vi "Agitator Module (Main).vi"(7 "Name of Parent Panel":string="Main.vi", 9 "New Center Coords":T1={"Horizontal"=470, "Vertical"=200}, 10 "Config":variant, 11 "Main UI Message Queue":refnum<queue>) -> ()   [LabVIEW 2018, in "Agitator Module.lvlib"]
doc: "This Continuous Measurement sample project is based on the Queued Message Handler template.\n\nThe Event Handling Loop generates messages based on user interface actions.\n\nThe Message Handling Loop processes messages generated by the Event Handling Loop, or by other messages. There are also Acquisition and Logging message handling loop subVIs, and a chart updating loop."
uses:
  Agitator Module.lvlib
  support/Message Queue/Message Cluster.ctl
  <vilib>/Utility/miscctls.llb/LVPoint32TypeDef.ctl
  controls/UI State.ctl
  Feed Module/Controls/Agitator Module Config Cluster.ctl
  Feed Module/Controls/Agitator Module Settings Cluster.ctl
  IKA EUROSTAR/IKA EUROSTAR Settings.ctl
  Feed Module/Controls/Agitator Module State Cluster.ctl
  Pump Module Folder/Measure Instrument/State Enum.ctl
  Sequencing/Squence Update Cluster.ctl
  Measure Instrument/State Enum.ctl
  Feed Module/Controls/Agitator Module Display.ctl
  support/Message Queue/Enqueue Message (Single).vi
  support/User Event - Stop/User Event - Stop.lvlib
  support/Message Queue/Message Queue.lvlib
  support/Support Library.lvlib
  Measure Instrument/Agitator Module Engine.lvlib
  Agitator Settings Dialog.vi
  support/Command Log VIs/Command Logging.lvlib
  Pump Module Folder/Measure Instrument/Pump Module Engine.lvlib
  Sequencing/Sequencing Library.lvlib
  Measure Instrument/Feed Module Engine.lvlib
  IKA EUROSTAR/IKA EUROSTAR.lvlib
panel:
  in  "Settings Button":bool
  out "H/W":dbl
  out "Original Height":u32
  out "Original Width":u32
  out "RPM":dbl format="%#_5f"
  out "Ring":u16(ring)=2
  out "ScanCode":i16
  out "Log File path":path
  out "Status":string
  in  "Exit":bool
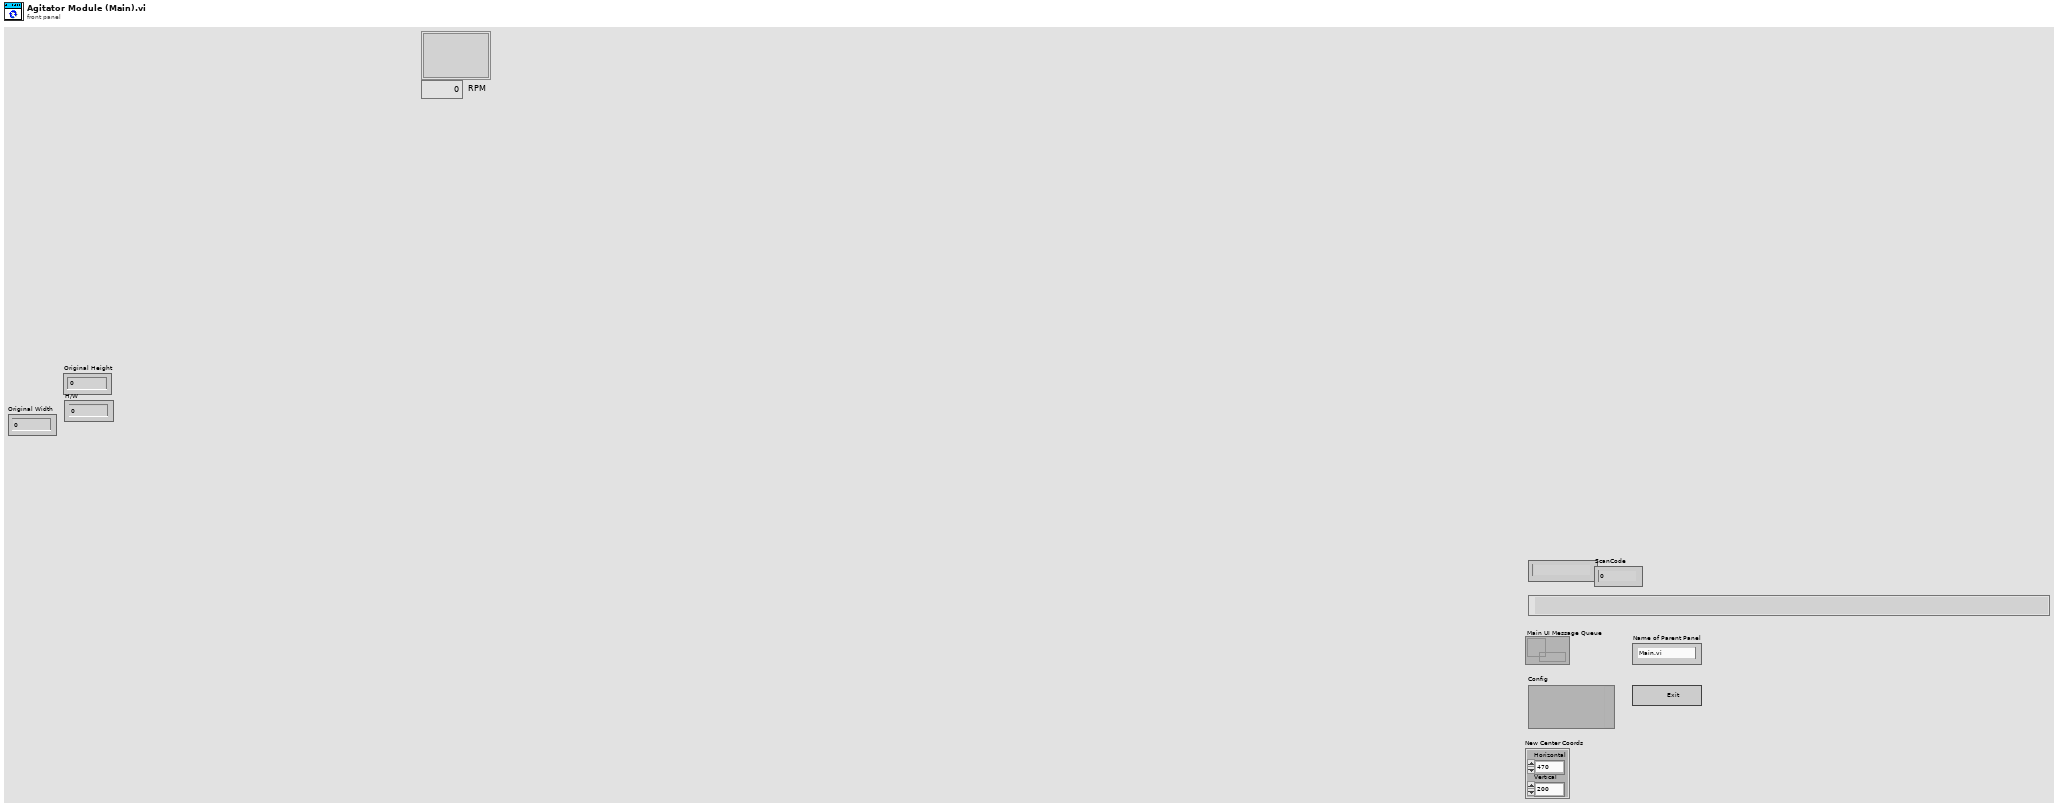
[diagram p1: front panel]
types:
  T1 = typedef "LVPoint32TypeDef.ctl" = cluster{"Horizontal":i32, "Vertical":i32}
  T2 = enum32{"Invalid", "Default", "Floating", "Floating/Auto-Hide", "Modal"}
  T3 = typedef "Agitator Module.lvlib/Agitator Module Config Cluster.ctl" = cluster{"GUID":string, "Drop Coords":T1, "Process Name":string, "User name":string, "Queue Name":string, "Settings":T4, "Load Count":i32}
  T4 = typedef "Agitator Module.lvlib/Agitator Module Settings Cluster.ctl" = cluster{"Cycle Period":dbl, "Agitator Type":string, "Setpoint (µm)":dbl, "IKA EUROSTAR Settings":T5}
  T5 = typedef "IKA EUROSTAR.lvlib/IKA EUROSTAR Settings.ctl" = cluster{"VISA resource name":refnum<visa-resource-name>, "Simulated?":bool}
  T6 = typedef "UI State.ctl" = enum16{"Idle", "Acquiring and Logging", "Waiting for Exit", "Waiting for Exit (Acq Stopped)", "Waiting for Exit (Log Stopped)", "Waiting for Stop", "Waiting for Stop (Acq Stopped)", "Waiting for Stop (Log Stopped)"}
  T7 = typedef "Agitator Module.lvlib/Agitator Module State Cluster.ctl" = cluster{"State":T8, "Start Time":timestamp, "Current Time":timestamp, "Agitator Module Config":T3, "Output Error":bool, "Log Started":bool, "First Iteration":bool, "Data":cluster{"Agitator rpm Value":dbl}, "Agitator On?":enum16{"Off", "On", "Not Initialized", "Over Cutoff"}}
  T8 = typedef "Pump Module.lvlib/Pump Module Engine.lvlib/State Enum.ctl" = enum16{"Measuring", "Idle", "Paused"}
  T9 = typedef "LVPointTypeDef.ctl" = cluster{"Horizontal":i16, "Vertical":i16}
  T10 = typedef "Agitator Module.lvlib/Agitator Message Queues.ctl" = cluster{"Agitator UI":refnum<queue>, "Agitator Engine":refnum<queue>, "Agitator Display":refnum<queue>}
  T11 = typedef "Sequencing Library.lvlib/Squence Update Cluster.ctl" = cluster{"Auto?":bool, "Manual Entry":dbl, "Setpoint":dbl}
  T12 = typedef "Feed Module.lvlib/Feed Module Engine.lvlib/State Enum.ctl" = enum16{"Measuring", "Idle", "Paused"}
  T13 = typedef "Agitator Module.lvlib/Agitator Module Display.ctl" = cluster{"Agitator On?":enum16{"Off", "On", "Not Initialized", "Over Cutoff"}, "Agitator RPM Value":dbl, "Cycle Period":dbl}
  T14 = enum16{"Off", "On", "Not Initialized", "Over Cutoff"}
  T15 = typedef "LVRectTypeDef.ctl" = cluster{"Left":i16, "Top":i16, "Right":i16, "Bottom":i16}
  T16 = cluster{"Shift":bool, "Ctrl":bool, "Alt":bool, "Cmd":bool, "Opt":bool}
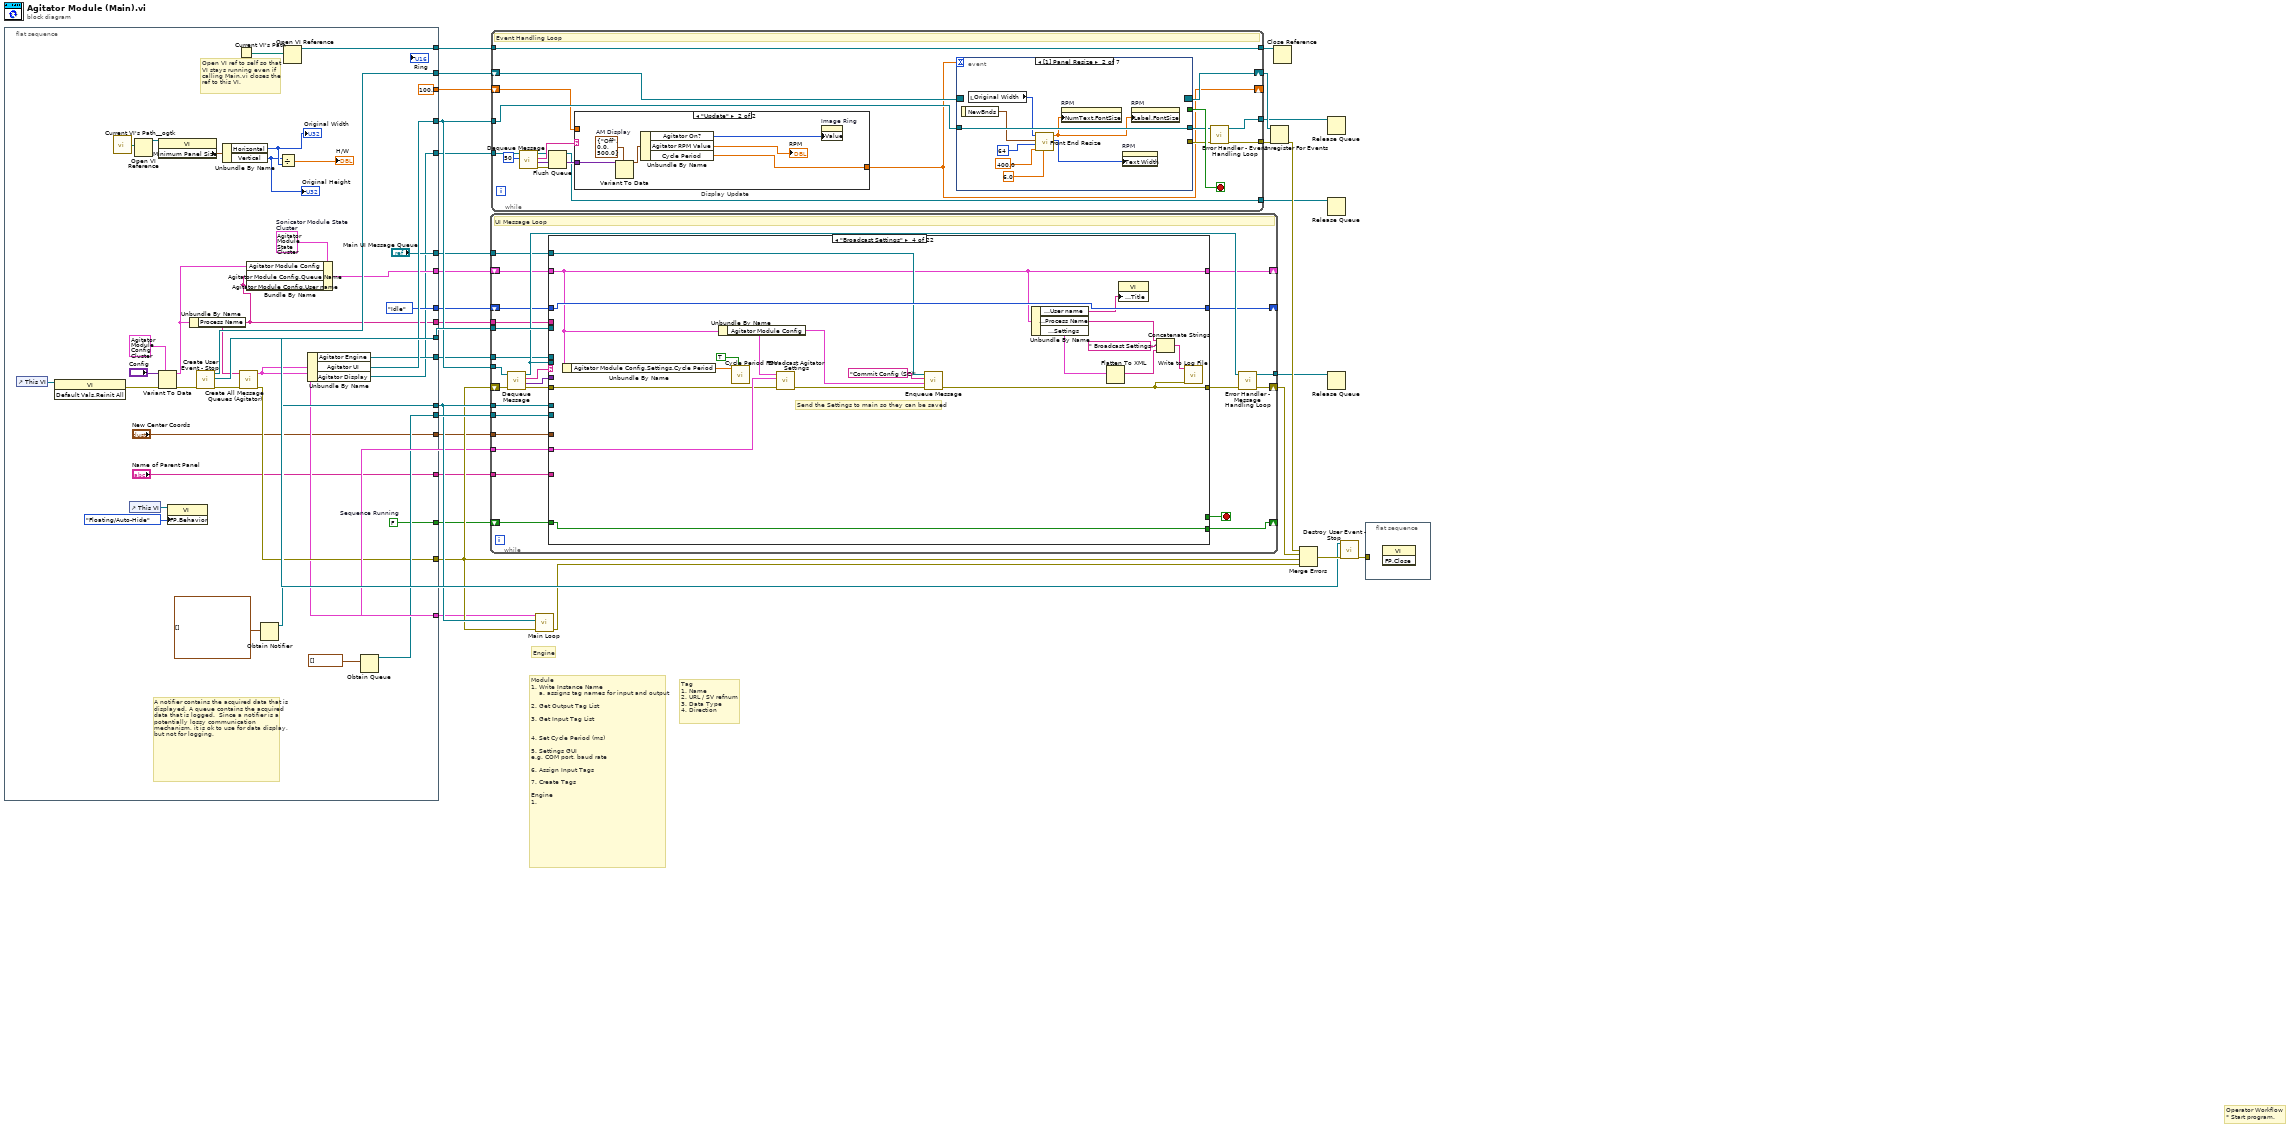
[diagram p0: block diagram]
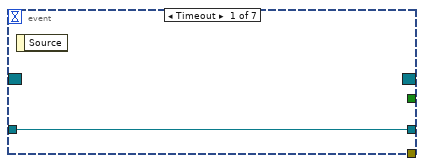
[diagram p3: hidden frame]
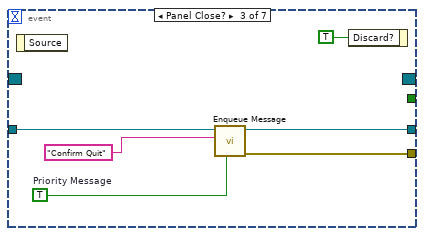
[diagram p4: hidden frame]
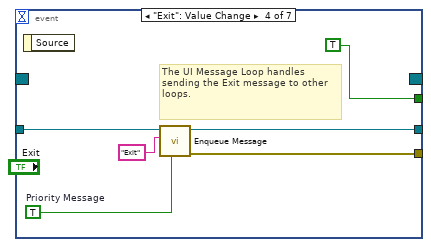
[diagram p5: hidden frame]
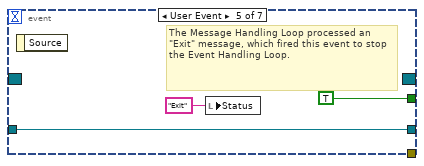
[diagram p6: hidden frame]
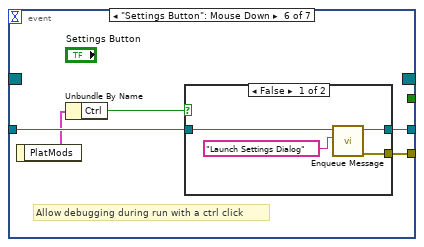
[diagram p7: hidden frame]
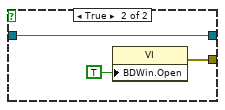
[diagram p8: hidden frame]
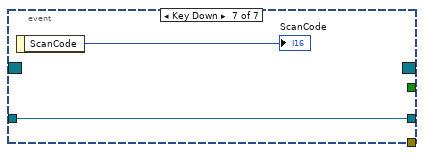
[diagram p9: hidden frame]
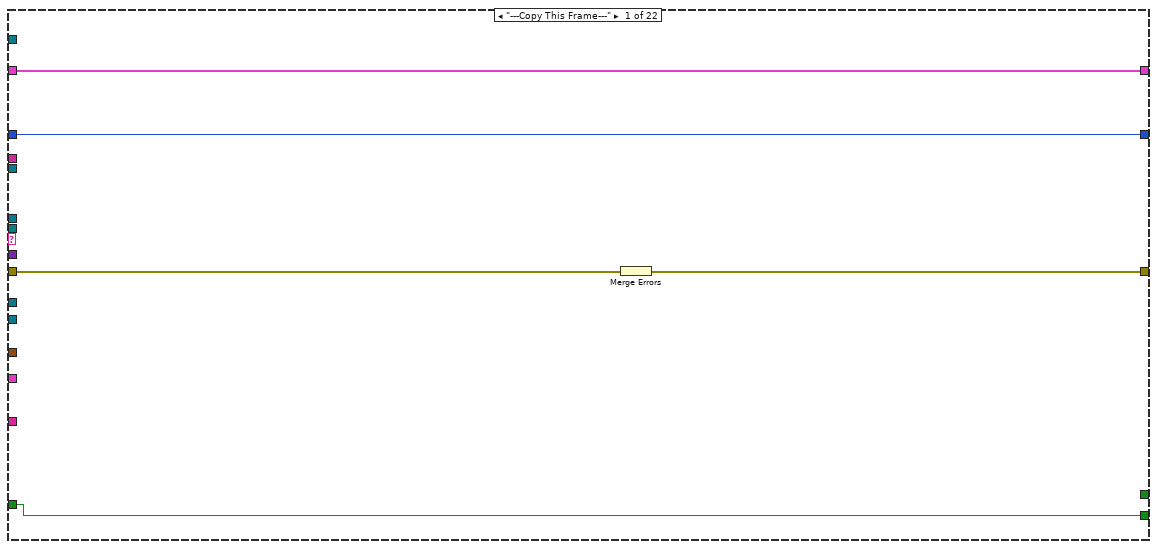
[diagram p10: hidden frame]
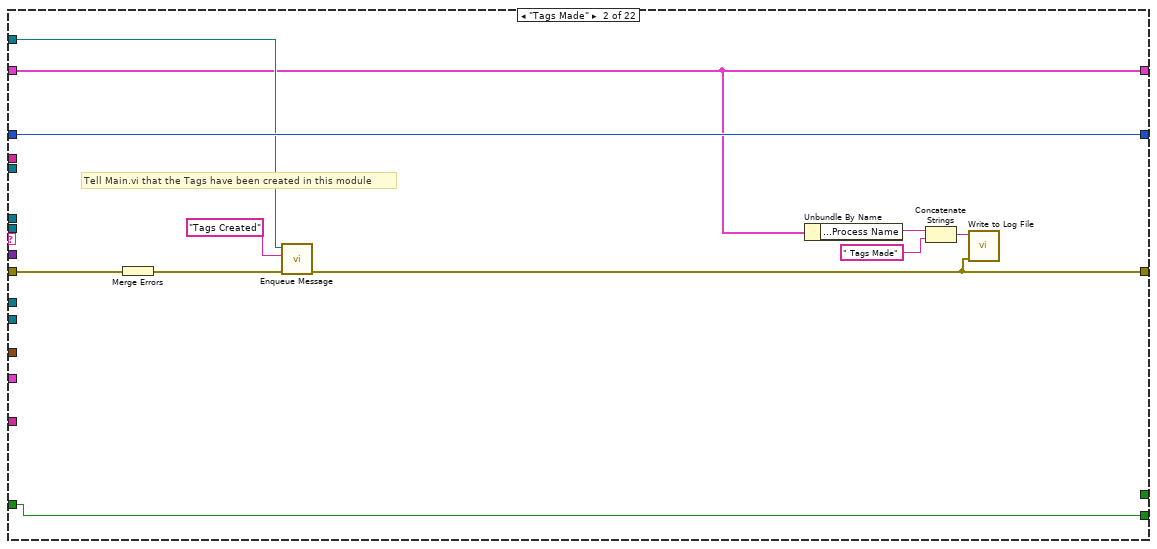
[diagram p11: hidden frame]
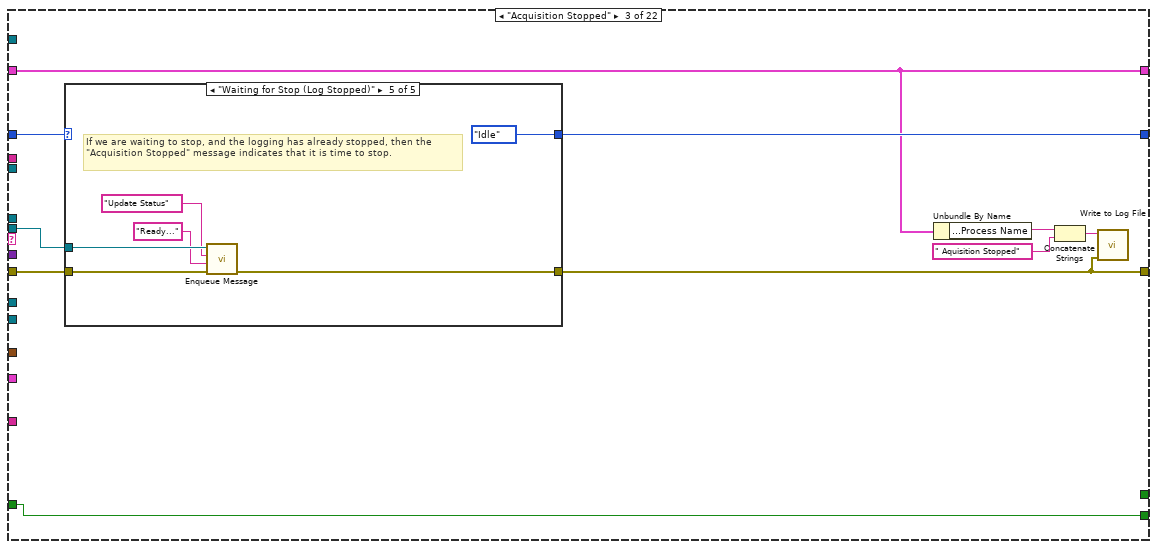
[diagram p12: hidden frame]
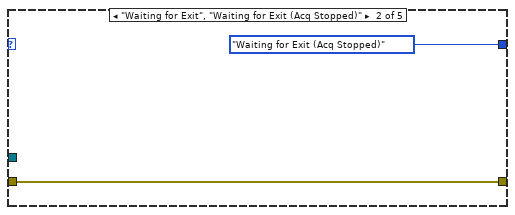
[diagram p14: hidden frame]
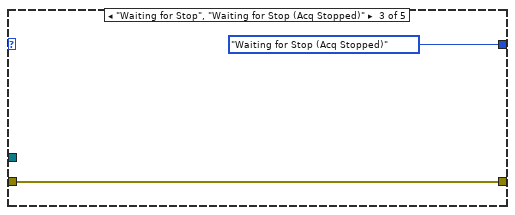
[diagram p15: hidden frame]
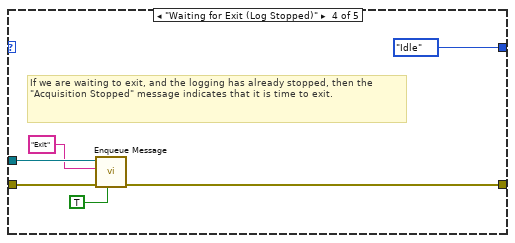
[diagram p16: hidden frame]
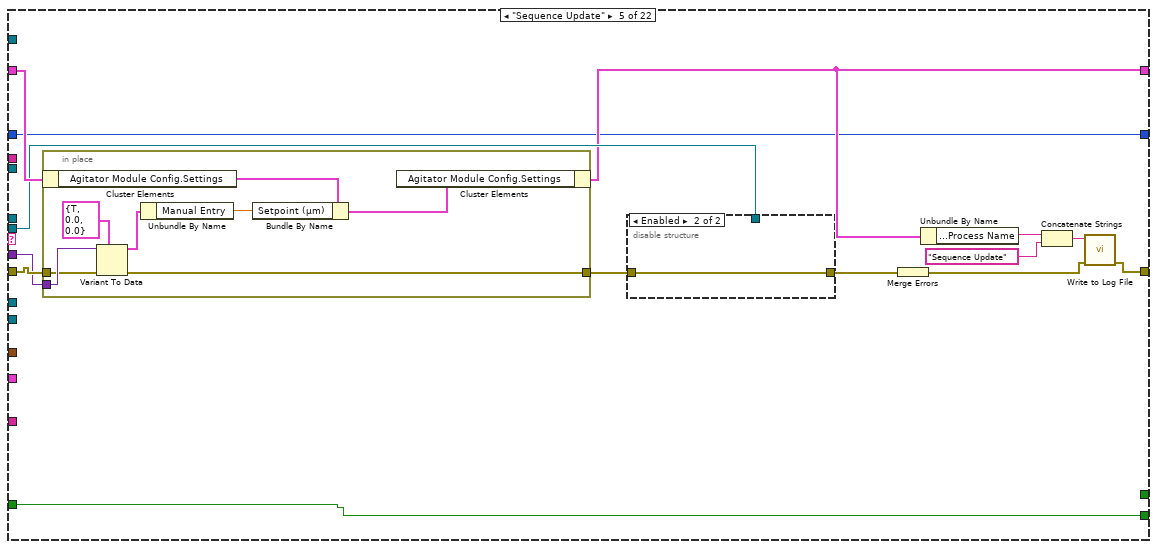
[diagram p17: hidden frame]
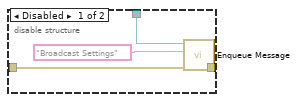
[diagram p18: hidden frame]
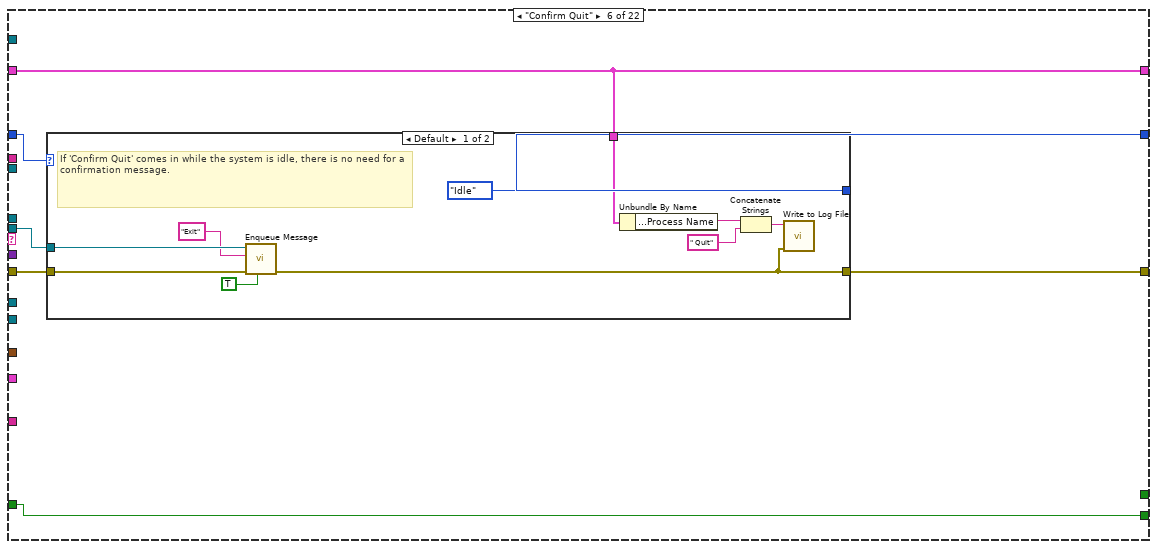
[diagram p19: hidden frame]
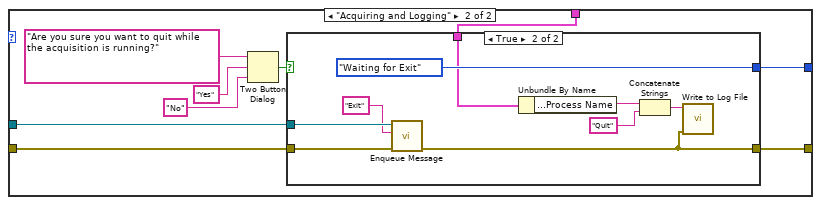
[diagram p20: hidden frame]
diagram:
  # "Engine"
  # "Operator Workflow\n* Start program."
  # "Module \n1. Write Instance Name\n    a. assigns tag names for input and output\n\n2. Get Output Tag List\n\n3. Get Input Tag List\n\n\n4. Set Cycle Period (ms)\n\n5. Settings GUI\ne.g. COM port, baud rate\n\n6. Assign Input Tags\n\n7. Create Tags\n\nEngine\n1."
  # "Tag\n1. Name\n2. URL / SV refnum\n3. Data Type\n4. Direction"
  n1 = flat-sequence {
    tunnel: [w66] -> w26
    tunnel: [w65] -> w25
    tunnel: [w64] -> w22
    tunnel: [UI_State."Idle" ("UI State")] -> w21
    tunnel: [w60] -> w20
    tunnel: [w59] -> w19
    tunnel: [w58] -> w17
    tunnel: [w57] -> w15
    tunnel: [w55] -> w14
    tunnel: ["Main UI Message Queue"] -> w13
    tunnel: [w50] -> w12
    tunnel: [w45] -> w11
    tunnel: [w44] -> w10
    tunnel: ["New Center Coords"] -> w9
    tunnel: ["Name of Parent Panel"] -> w8
    tunnel: [100.0 ("Cycle Period")] -> w6
    tunnel: [w37] -> w2
    tunnel: [w36] -> w1
    frame #0 {
      w37 = FALSE  # Sequence Running
      w51 = T7 {"State"=enum."Idle", "Start Time"=timestamp(0 s since 1904-01-01), "Current Time"=timestamp(0 s since 1904-01-01), "Agitator Module Config"={"GUID"="PID1-Mettler Toledo Scale 1", "Drop Coords"={"Horizontal"=0, "Vertical"=0}, "Process Name"="PID1-Setpoint", "User name"="", "Queue Name"="", "Settings"={"Cycle Period"=500.0, "Agitator Type"="", "Setpoint (µm)"=0.0, "IKA EUROSTAR Settings"={"VISA resource name"="", "Simulated?"=FALSE}}, "Load Count"=0}, "Output Error"=FALSE, "Log Started"=FALSE, "First Iteration"=FALSE, "Data"={"Agitator rpm Value"=0.0}, "Agitator On?"=enum."Off"}  # Sonicator Module State Cluster
      # "Open VI ref to self so that\nVI stays running even if\ncalling Main.vi closes the\nref to this VI."
      # "A notifier contains the acquired data that is displayed. A queue contains the acquired data that is logged.  Since a notifier is a potentially lossy communication mechanism, it is ok to use for data display, but not for logging."
      n2 = control-ref of="This VI"() -> (w48:refnum<vi>)
      n3 = invoke class="VI" method="Default Vals.Reinit All"(reference=w48) -> (error out=w41:errorcluster)  [unwired: 2 in, 2 out]
      n4 = call <userlib>:"Current VI's Path__ogtk.vi"() -> ("Current VI's Path (+ Relative)"=w34:path)  [unwired: 1 in]
      n5 = control-ref of="This VI"() -> (w39:refnum<vi>)
      n6 = Open VI Reference(vi path=w34) -> (vi reference=w33:refnum<vi>)  [unwired: 5 in, 1 out]
      n7 = Variant To Data(error in=w41, type=T3 {"GUID"="", "Drop Coords"={"Horizontal"=0, "Vertical"=0}, "Process Name"="", "User name"="", "Queue Name"="", "Settings"={"Cycle Period"=500.0, "Agitator Type"="", "Setpoint (µm)"=0.0, "IKA EUROSTAR Settings"={"VISA resource name"="", "Simulated?"=FALSE}}, "Load Count"=0} ("Feed Module Config"), Variant="Config") -> (data=w49:T3, error out=w54:errorcluster)
      n8 = property class="VI"(reference=w33) -> ("Minimum Panel Size"=w32:T9)  [unwired: 1 in, 2 out]
      n9 = property class="VI"(reference=w39, "FP.Behavior"=T2."Floating/Auto-Hide" ("Front Panel Window:Behavior")) -> ()  [unwired: 1 in, 2 out]
      n10 = Unbundle By Name(w49) -> ("Process Name"=w36:string)
      n11 = call "Create User Event - Stop.vi"("error in (no error)"=w54) -> ("error out"=w46:errorcluster, "User Event - Stop"=w65:refnum<user-event>, "Stop Event Registration Refnum"=w66:refnum<event-registration>)  [unwired: 8 in]
      n12 = Unbundle By Name(w32) -> ("Horizontal"=w31:i16, "Vertical"=w30:i16)
      "Original Width" <- w31
      "Original Height" <- w30
      n13 = Current VI's Path() -> (path=w56:path)
      n14 = call "Create All Message Queues (Agitator).vi"("error in (no error)"=w46, "Process Name"=w36) -> ("error out"=w45:errorcluster, "Message Queues"=w44:T10)  [unwired: 8 in]
      n15 = Bundle By Name(cluster=w51, "Agitator Module Config"=w49, "Agitator Module Config.Queue Name"=w36, "Agitator Module Config.User name"=w36) -> (w55:T7)
      n16 = Obtain Notifier(notification data type=waveform(dbl)[] []) -> (notifier out=w58:refnum<notifier>)  [unwired: 3 in, 2 out]
      n17 = Divide(x=w30, y=w31) -> (x/y=→"H/W":dbl)
      n18 = Open VI Reference(vi path=w56) -> (vi reference=w57:refnum<vi>)  [unwired: 5 in, 1 out]
      n19 = Unbundle By Name(w44) -> ("Agitator Engine"=w60:refnum<queue>, "Agitator UI"=w64:refnum<queue>, "Agitator Display"=w50:refnum<queue>)
      n20 = Obtain Queue(element data type=waveform(dbl)[] []) -> (queue out=w59:refnum<queue>)  [unwired: 4 in, 2 out]
    }
  }
  n21 = while {
    tunnel: w22 -> [w86]
    tunnel: w25 -> [w90]
    shift-right: [w82] -> w29
    shift-left: w11 -> [w89]
    shift-right: [w73] -> _
    shift-left: w14 -> [w75]
    tunnel: w17 -> [w85]
    tunnel: w19 -> [w84]
    shift-right: [w79] -> _
    shift-left: w21 -> [w80]
    tunnel: w20 -> [w78]
    tunnel: w10 -> [w77]
    tunnel: w13 -> [w74]
    tunnel: w1 -> [w72]
    tunnel: w9 -> [w71]
    tunnel: w8 -> [w70]
    tunnel: [w69] -> w3
    shift-right: [w67] -> _
    shift-left: w2 -> [w68]
    stop <- w91 stop-if-true
    # "UI Message Loop"
    n22 = call "Dequeue Message.vi"("error in (no error)"=w89, "Message Queue"=w86) -> ("error out"=w76:errorcluster, "Message Data"=w87:variant, "Message"=w88:string, "dup Message Queue"=w81:refnum<queue>)  [unwired: 6 in]
    n23 = case "Message Cases" shown="\"Broadcast Settings\"" w88 {
      selector: w88 -> [_ _ _ _ _ _ _ _ _ _ _ _ _ _ _ _ _ _ _ _ _ w470]
      tunnel: w81 -> [_ _ w114 _ w157 w186 _ w238 w253 w276 _ w317 _ w343 _ w383 w387 _ _ w456 _ _]
      tunnel: w76 -> [w96 w107 w115 w149 w161 w185 w221 w233 w257 w275 w302 w313 w333 w344 w368 w382 w388 w411 w425 w451 w466 _]
      tunnel: [w95 w98 w110 w142 w160 w184 w222 w228 w244 w260 w302 w305 w332 w339 w371 w378 w391 w418 w427 w443 w467 w469] -> w83
      tunnel: [_ _ _ _ _ _ _ _ _ TRUE _ _ _ _ _ _ _ _ _ _ _ _] -> w91
      tunnel: w87 -> [_ _ _ _ w158 _ w224 _ w256 w265 _ _ _ _ w369 _ _ _ _ _ w465 _]
      tunnel: w90 -> [_ _ _ _ _ _ _ _ _ w286 _ _ _ _ _ _ _ _ _ _ _ _]
      tunnel: w75 -> [w93 w99 w109 w141 w159 w182 w219 w227 w243 w259 w299 w304 w328 w338 w375 w377 w394 w412 w426 w442 w460 w475]
      tunnel: w85 -> [_ _ _ _ _ _ _ _ _ w284 _ _ _ _ _ _ _ _ _ _ _ _]
      tunnel: w84 -> [_ _ _ _ _ _ _ _ _ w280 _ _ _ _ _ _ _ _ _ _ _ _]
      tunnel: w80 -> [w94 w106 w117 w153 w155 w187 w220 w234 w248 w273 _ _ w334 w346 w374 _ _ _ _ w452 w461 w479]
      tunnel: [w94 w106 w116 w153 w155 w183 w220 w235 w248 w272 UI_State."Idle" ("UI State") UI_State."Idle" ("UI State") w334 w345 w374 UI_State."Acquiring and Logging" ("UI State") UI_State."Acquiring and Logging" ("UI State") UI_State."Acquiring and Logging" ("UI State") UI_State."Acquiring and Logging" ("UI State") w453 w461 w479] -> w79
      tunnel: w78 -> [_ _ _ _ _ _ _ _ _ w279 _ _ _ _ _ _ _ w416 w434 w450 _ _]
      tunnel: w77 -> [_ _ _ w152 _ _ _ _ _ _ _ _ w325 _ _ _ _ _ _ _ _ _]
      tunnel: w74 -> [_ w103 _ w146 _ _ _ _ _ w264 _ _ _ _ _ _ _ _ _ _ _ _]
      tunnel: [w93 w99 w109 w141 w156 w182 w219 w227 w243 w259 w299 w304 w326 w338 w375 w377 w393 w412 w426 w442 w460 w475] -> w73
      tunnel: w72 -> [_ _ _ _ _ _ _ _ _ _ _ w311 _ _ _ _ _ _ _ _ _ _]
      tunnel: w71 -> [_ _ _ _ _ _ _ _ _ _ _ w310 _ _ _ _ _ _ _ _ _ _]
      tunnel: w70 -> [_ _ _ _ _ _ _ _ _ _ _ w309 _ _ _ _ _ _ _ _ _ _]
      tunnel: w68 -> [w92 w97 w108 w137 w154 w181 w218 w226 w241 w258 w298 w303 w327 w337 w365 w376 w389 w410 w424 w441 w459 w468]
      tunnel: [w92 w97 w108 w137 w154 w181 w218 w226 w241 w258 w298 w303 w327 w337 w365 w376 w390 w410 w424 w441 w459 w468] -> w67
      frame "---Copy This Frame---" {
        # "Duplicate this frame when creating new messages.  Change this comment in the duplicated frame to describe this message."
        n24 = Merge Errors(w96) -> (w95:errorcluster)
      }
      frame "Tags Made" {
        # "Tell Main.vi that the Tags have been created in this module"
        # "Duplicate this frame when creating new messages.  Change this comment in the duplicated frame to describe this message."
        n25 = Merge Errors(w107) -> (w104:errorcluster)
        n26 = call-poly "Enqueue Message.vi"("error in (no error)"=w104, "Message"="Tags Created", "Message Queue"=w103) -> ("error out"=w98:errorcluster)  [unwired: 7 in, 1 out]
        n27 = Unbundle By Name(w99) -> ("Agitator Module Config.Process Name"=w102:string)
        n28 = Concatenate Strings(w102, " Tags Made" ("text")) -> (w100:string)
        n29 = call "Write to Log File.vi"("error in"=w98, "text"=w100) -> ()  [unwired: 9 in, 1 out]
      }
      frame "Acquisition Stopped" {
        # "Logic for determining what action to take when the acquisition has stopped."
        n30 = case shown="\"Waiting for Stop (Log Stopped)\"" w117 {
          selector: w117 -> [w119 _ _ _ _]
          tunnel: [w119 UI_State."Waiting for Exit (Acq Stopped)" ("UI State") UI_State."Waiting for Stop (Acq Stopped)" ("UI State") UI_State."Idle" ("UI State") UI_State."Idle" ("UI State")] -> w116
          tunnel: w115 -> [w118 w120 w122 w128 w134]
          tunnel: [w118 w120 w122 w127 w133] -> w110
          tunnel: w114 -> [_ _ _ w126 w132]
          frame Default {
          }
          frame "Waiting for Exit", "Waiting for Exit (Acq Stopped)" {
          }
          frame "Waiting for Stop", "Waiting for Stop (Acq Stopped)" {
          }
          frame "Waiting for Exit (Log Stopped)" {
            # "If we are waiting to exit, and the logging has already stopped, then the \"Acquisition Stopped\" message indicates that it is time to exit."
            n31 = call-poly "Enqueue Message.vi"("Priority Message? (F)"=TRUE, "error in (no error)"=w128, "Message"="Exit", "Message Queue"=w126) -> ("error out"=w127:errorcluster)  [unwired: 6 in, 1 out]
          }
          frame "Waiting for Stop (Log Stopped)" {
            # "If we are waiting to stop, and the logging has already stopped, then the \"Acquisition Stopped\" message indicates that it is time to stop."
            n32 = call-poly "Enqueue Message.vi"("error in (no error)"=w134, "Message Data"="Ready..." ("Message"), "Message"="Update Status", "Message Queue"=w132) -> ("error out"=w133:errorcluster)  [unwired: 6 in, 1 out]
          }
        }
        n33 = Unbundle By Name(w109) -> ("Agitator Module Config.Process Name"=w113:string)
        n34 = Concatenate Strings(w113, " Aquisition Stopped" ("text")) -> (w111:string)
        n35 = call "Write to Log File.vi"("error in"=w110, "text"=w111) -> ()  [unwired: 9 in, 1 out]
      }
      frame "Broadcast Settings" {
        # "Send the Settings to main so they can be saved"
        # "Send the 'Update Settings' message to the Logging and Acquisition message loops."
        n36 = Unbundle By Name(w141) -> ("Agitator Module Config.Settings.Cycle Period"=w150:dbl)
        n37 = Unbundle By Name(w141) -> ("Agitator Module Config"=w145:T3)
        n38 = call "Cycle Period FGV.vi"("Write"=TRUE, "Cycle Period In (ms)"=w150) -> ()  [unwired: 8 in, 2 out]
        n39 = call "Broadcast Agitator Settings.vi"("error in (no error)"=w149, "Message Queues"=w152, "Agitator Module Config"=w145) -> ("error out"=w147:errorcluster)  [unwired: 8 in]
        n40 = call-poly "Enqueue Message.vi"("error in (no error)"=w147, "Message Data"=w145, "Message"="Commit Config (SC)", "Message Queue"=w146) -> ("error out"=w142:errorcluster)  [unwired: 6 in, 1 out]
        n41 = Unbundle By Name(w141) -> ("Agitator Module Config.User name"=w136:string, "Agitator Module Config.Process Name"=w138:string, "Agitator Module Config.Settings"=w140:T4)
        n42 = Flatten To XML(anything=w140) -> (xml string=w139:string)
        n43 = property class="VI"("Front Panel.Title"=w136) -> ()  [unwired: 2 in, 2 out]
        n44 = Concatenate Strings(w138, " Broadcast Settings: " ("text"), w139) -> (w143:string)
        n45 = call "Write to Log File.vi"("error in"=w142, "text"=w143) -> ()  [unwired: 9 in, 1 out]
      }
      frame "Sequence Update" {
        n46 = in-place {
          in-place-border: w158 -> [w177]
          in-place-border: w161 -> [w176]
          in-place-border: [w175] -> w166
          n47 = in-place-cluster #1(w159) -> ("Agitator Module Config.Settings"=w173:T4)
          n48 = Variant To Data(error in=w176, type=T11 {"Auto?"=TRUE, "Manual Entry"=0.0, "Setpoint"=0.0} ("Cluster"), Variant=w177) -> (data=w179:T11, error out=w175:errorcluster)
          n49 = Unbundle By Name(w179) -> ("Manual Entry"=w178:dbl)
          n50 = Bundle By Name(cluster=w173, "Setpoint (µm)"=w178) -> (w174:T4)
          n51 = in-place-cluster #1("Agitator Module Config.Settings"=w174) -> (w156:T7)
        }
        n52 = disable-structure shown="Enabled" {
          disable-tunnel: [w171 w172] -> w167
          disable-tunnel: w157 -> [w169 _]
          disable-tunnel: w166 -> [w168 w172]
          frame Disabled {
            n53 = call-poly "Enqueue Message.vi"("error in (no error)"=w168, "Message"="Broadcast Settings", "Message Queue"=w169) -> ("error out"=w171:errorcluster)  [unwired: 7 in, 1 out]
          }
          frame Enabled {
          }
        }
        n54 = Merge Errors(w167) -> (w163:errorcluster)
        n55 = Unbundle By Name(w156) -> ("Agitator Module Config.Process Name"=w165:string)
        n56 = Concatenate Strings(w165, "Sequence Update" ("text")) -> (w162:string)
        n57 = call "Write to Log File.vi"("error in"=w163, "text"=w162) -> ("error out"=w160:errorcluster)  [unwired: 9 in]
      }
      frame "Confirm Quit" {
        # "Confirm Quit - Message that can confirm whether or not the user wants to exit the application."
        n58 = case shown="Default" w187 {
          tunnel: w186 -> [w196 w203]
          tunnel: w185 -> [w195 w201]
          tunnel: [w189 w200] -> w184
          tunnel: [UI_State."Idle" ("UI State") w199] -> w183
          tunnel: w182 -> [w188 w198]
          frame Default {
            # "If 'Confirm Quit' comes in while the system is idle, there is no need for a confirmation message."
            n59 = call-poly "Enqueue Message.vi"("Priority Message? (F)"=TRUE, "error in (no error)"=w195, "Message"="Exit", "Message Queue"=w196) -> ("error out"=w189:errorcluster)  [unwired: 6 in, 1 out]
            n60 = Unbundle By Name(w188) -> ("Agitator Module Config.Process Name"=w192:string)
            n61 = Concatenate Strings(w192, " Quit" ("text")) -> (w190:string)
            n62 = call "Write to Log File.vi"("error in"=w189, "text"=w190) -> ()  [unwired: 9 in, 1 out]
          }
          frame "Acquiring and Logging" {
            n63 = Two Button Dialog(message="Are you sure you want to quit while the acquisition is running?" ("Confirm Quit Message"), 1:"No" ("No"), 2:"Yes" ("Yes")) -> (T button?=w202:bool)
            n64 = case shown="True" w202 {
              tunnel: w203 -> [_ w217]
              tunnel: w201 -> [w207 w216]
              tunnel: [w207 w210] -> w200
              tunnel: [UI_State."Acquiring and Logging" ("UI State") UI_State."Waiting for Exit" ("UI State")] -> w199
              tunnel: w198 -> [_ w209]
              frame False {
                # "User did not want to quit."
              }
              frame True {
                n65 = call-poly "Enqueue Message.vi"("error in (no error)"=w216, "Message"="Exit", "Message Queue"=w217) -> ("error out"=w210:errorcluster)  [unwired: 7 in, 1 out]
                n66 = Unbundle By Name(w209) -> ("Agitator Module Config.Process Name"=w213:string)
                n67 = Concatenate Strings(w213, "Quit" ("text")) -> (w211:string)
                n68 = call "Write to Log File.vi"("error in"=w210, "text"=w211) -> ()  [unwired: 9 in, 1 out]
              }
            }
          }
        }
      }
      frame "Display Log File Path" {
        n69 = Variant To Data(error in=w221, type=path "", Variant=w224) -> (data=→"Log File path":path, error out=w222:errorcluster)
      }
      frame "E-Stop" {
        # "E-Stop has no effect on the scale"
        # "Message Acquisition and Logging loops to stop"
        # "Stop the pumps."
        n70 = call-poly "Enqueue Message.vi"("error in (no error)"=w233, "Message Data"="Ready..." ("Ready..."), "Message"="Update Status", "Message Queue"=w238) -> ("error out"=w232:errorcluster)  [unwired: 6 in, 1 out]
        n71 = case shown="\"Waiting for Exit\"" w234 {
          selector: w234 -> [_ w240]
          tunnel: [UI_State."Waiting for Stop" ("UI State") w240] -> w235
          frame Default {
          }
          frame "Waiting for Exit" {
          }
        }
        n72 = Merge Errors(w232) -> (w228:errorcluster)
        n73 = Unbundle By Name(w227) -> ("Agitator Module Config.Process Name"=w231:string)
        n74 = Concatenate Strings(w231, " E-STOP" ("text")) -> (w229:string)
        n75 = call "Write to Log File.vi"("error in"=w228, "text"=w229) -> ()  [unwired: 9 in, 1 out]
      }
      frame "Error" {
        # "Error - Check the error message data and respond accordingly. This message is sent by the \"Error Handler\" VIs at the end of each loop in this application."
        n76 = Variant To Data(error in=w257, type=errorcluster {"status"=FALSE, "code"=0, "source"=""} ("error out"), Variant=w256) -> (data=w254:errorcluster, error out=w250:errorcluster)
        n77 = call <vilib>:"General Error Handler.vi"("error in (no error)"=w254) -> ("message"=w242:string)  [unwired: 10 in, 4 out]
        n78 = call-poly "Enqueue Message.vi"("Priority Message? (F)"=TRUE, "Message"="Exit", "Message Queue"=w253) -> ("error out"=w249:errorcluster)  [unwired: 7 in, 1 out]
        n79 = Merge Errors(w249, w250) -> (w244:errorcluster)
        n80 = Unbundle By Name(w243) -> ("Agitator Module Config.Process Name"=w247:string)
        n81 = Concatenate Strings(w247, " Error: " ("text"), w242) -> (w245:string)
        n82 = call "Write to Log File.vi"("error in"=w244, "text"=w245) -> ()  [unwired: 9 in, 1 out]
      }
      frame "Exit" {
        w268 = TRUE  # Delete Module?
        # "Don't check the error outs. The acquisition and logging queues may have already been released."
        # "Close references owned by the Main VI."
        # "Stop the VI"
        # "Exit - Fire the User Event to stop the Event Handling Loop.  Also send Exit messages to the Acquisition and Logging loops."
        n83 = call "Fire User Event - Stop.vi"("User Event - Stop"=w286) -> ("error out"=w285:errorcluster)  [unwired: 10 in]
        n84 = Build Array(w279) -> (w278:refnum<queue>[])
        n85 = for {
          tunnel: w278 -> [w295] mode=indexing
          n86 = call-poly "Enqueue Message.vi"("Message"="Stop", "Message Queue"=w295) -> ("dup Message Queue"=w296:refnum<queue>)  [unwired: 8 in, 1 out]
          n87 = call-poly "Enqueue Message.vi"("Message"="Exit", "Message Queue"=w296) -> ()  [unwired: 8 in, 2 out]
        }
        n88 = Variant To Data(type=w268, Variant=w265) -> (data=w267:bool, error out=w269:errorcluster)  [unwired: 1 in]
        n89 = call-poly "Enqueue Message.vi"("error in (no error)"=w275, "Message Data"="Ready..." ("Ready..."), "Message"="Update Status", "Message Queue"=w276) -> ("error out"=w274:errorcluster, "dup Message Queue"=w271:refnum<queue>)  [unwired: 6 in]
        n90 = Select(t=w268, s=w269, f=w267) -> (s? t:f=w266:bool)
        n91 = case "Don't enqueue Delete Module if opening campaign because it\nwill already have been deleted and new config loaded and we create\na race condition." shown="True" w266 {
          tunnel: w264 -> [_ w290]
          tunnel: w259 -> [_ w289]
          frame False {
          }
          frame True {
            n92 = Unbundle By Name(w289) -> ("Agitator Module Config.GUID"=w288:string)
            n93 = call-poly "Enqueue Message.vi"("Message Data"=w288, "Message"="Delete Module", "Message Queue"=w290) -> ()  [unwired: 7 in, 2 out]
          }
        }
        n94 = Release Queue(queue=w271, error in (no error)=w274) -> (error out=w283:errorcluster)  [unwired: 1 in, 2 out]
        n95 = Release Notifier(notifier=w284, error in (no error)=w283) -> (error out=w282:errorcluster)  [unwired: 1 in, 2 out]
        n96 = Release Queue(queue=w280, error in (no error)=w282) -> (error out=w281:errorcluster)  [unwired: 1 in, 2 out]
        n97 = Merge Errors(w285, w281) -> (w260:errorcluster)
        n98 = case shown="Default" w273 {
          selector: w273 -> [_ w293]
          tunnel: [UI_State."Waiting for Stop" ("UI State") w293] -> w272
          frame Default {
          }
          frame "Waiting for Exit" {
          }
        }
        n99 = Unbundle By Name(w259) -> ("Agitator Module Config.Process Name"=w263:string)
        n100 = Concatenate Strings(w263, " Exit" ("text")) -> (w261:string)
        n101 = call "Write to Log File.vi"("error in"=w260, "text"=w261) -> ()  [unwired: 9 in, 1 out]
      }
      frame "Init UI Refs" {
        # "Init UI Refs - Store control references for UI controls.  Also enable/disable controls appropriately."
        n102 = property class="VI"("Front Panel.Closeable"=TRUE ("Front Panel Window:Closeable")) -> ()  [unwired: 2 in, 2 out]
      }
      frame "Initialize" {
        # "Initialize - Get configuration settings, then message the UI to initialize, and broadcast the settings to the other message loops."
        n103 = call-poly "Enqueue Message.vi"("error in (no error)"=w313, "Message"="Init UI Refs", "Message Queue"=w317) -> ("error out"=w315:errorcluster, "dup Message Queue"=w316:refnum<queue>)  [unwired: 7 in]
        n104 = property class="VI" props=["FP.State"]() -> (reference out=w312:refnum<vi>)  [unwired: 2 in, 2 out]
        n105 = call "Make Child and Move.vi"("Process Name"=w311, "Name of Parent Panel"=w309, "New Center Coords"=w310, "VI in"=w312) -> ()  [unwired: 8 in]
        n106 = call-poly "Enqueue Message.vi"("error in (no error)"=w315, "Message"="Broadcast Settings", "Message Queue"=w316) -> ("error out"=w323:errorcluster, "dup Message Queue"=w322:refnum<queue>)  [unwired: 7 in]
        n107 = call-poly "Enqueue Message.vi"("error in (no error)"=w323, "Message Data"="Ready..." ("Ready..."), "Message"="Update Status", "Message Queue"=w322) -> ("error out"=w305:errorcluster)  [unwired: 6 in, 1 out]
        n108 = Unbundle By Name(w304) -> ("Agitator Module Config.Process Name"=w308:string)
        n109 = Concatenate Strings(w308, " Initialize" ("text")) -> (w306:string)
        n110 = call "Write to Log File.vi"("error in"=w305, "text"=w306) -> ()  [unwired: 9 in, 1 out]
      }
      frame "Launch Settings Dialog" {
        # "Launch the Settings Dialog when the user clicks the 'Settings' button."
        n111 = in-place {
          n112 = in-place-cluster #2(w328) -> ("Agitator Module Config.Load Count"=w335:i32)
          n113 = Increment(x=w335) -> (x+1=w336:i32)
          n114 = in-place-cluster #2("Agitator Module Config.Load Count"=w336) -> (w324:T7)
        }
        n115 = call-by-ref "?"("error in (no error)"=w333, "Message Queues"=w325, "Agitator Module State Cluster In"=w324) -> ("error out"=w332:errorcluster, "Agitator Module State Cluster Out"=w326:T7)  [unwired: 7 in, 4 out]
        n116 = Unbundle By Name(w326) -> ("Agitator Module Config.Process Name"=w331:string)
        n117 = Concatenate Strings(w331, " Setting Dialog Launched" ("text")) -> (w329:string)
        n118 = call "Write to Log File.vi"("error in"=w332, "text"=w329) -> ()  [unwired: 9 in, 1 out]
      }
      frame "Logging Stopped" {
        # "Logic for determining what action to take when the logging has stopped."
        n119 = case shown="\"Waiting for Exit (Acq Stopped)\"" w346 {
          selector: w346 -> [w348 _ _ _ _]
          tunnel: [w348 UI_State."Waiting for Exit (Log Stopped)" ("UI State") UI_State."Waiting for Stop (Log Stopped)" ("UI State") UI_State."Idle" ("UI State") UI_State."Idle" ("UI State")] -> w345
          tunnel: w344 -> [w347 w349 w351 w357 w363]
          tunnel: [w347 w349 w351 w356 w362] -> w339
          tunnel: w343 -> [_ _ _ w355 w361]
          frame Default {
          }
          frame "Waiting for Exit", "Waiting for Exit (Log Stopped)" {
          }
          frame "Waiting for Stop", "Waiting for Stop (Log Stopped)" {
          }
          frame "Waiting for Exit (Acq Stopped)" {
            # "If we are waiting to exit, and the acquisition has already stopped, then the \"Logging Stopped\" message indicates that it is time to exit."
            n120 = call-poly "Enqueue Message.vi"("Priority Message? (F)"=TRUE, "error in (no error)"=w357, "Message"="Exit", "Message Queue"=w355) -> ("error out"=w356:errorcluster)  [unwired: 6 in, 1 out]
          }
          frame "Waiting for Stop (Acq Stopped)" {
            # "If we are waiting to stop, and the acquisition has already stopped, then the \"Logging Stopped\" message indicates that it is time to stop."
            n121 = call-poly "Enqueue Message.vi"("error in (no error)"=w363, "Message Data"="Ready..." ("Message"), "Message"="Update Status", "Message Queue"=w361) -> ("error out"=w362:errorcluster)  [unwired: 6 in, 1 out]
          }
        }
        n122 = Unbundle By Name(w338) -> ("Agitator Module Config.Process Name"=w342:string)
        n123 = Concatenate Strings(w342, " Logging Stopped" ("text")) -> (w340:string)
        n124 = call "Write to Log File.vi"("error in"=w339, "text"=w340) -> ()  [unwired: 9 in, 1 out]
      }
      frame "Send to Sequence" {
        n125 = Variant To Data(error in=w368, type=refnum<queue> refnum ("Message Queue"), Variant=w369) -> (data=w366:refnum<queue>, error out=w367:errorcluster)
        n126 = local read "RPM"() -> (w372:dbl)
        n127 = call-poly "Enqueue Message.vi"("error in (no error)"=w367, "Message Data"=w372, "Message"="Sent to Sequence", "Message Queue"=w366) -> ("error out"=w371:errorcluster)  [unwired: 6 in, 1 out]
      }
      frame "Start" {
        # "Message Acquisition and Logging loops to start"
        # "Start - Enable/Disable buttons appropriately for an acquisition that has started, and update status display."
        n128 = call-poly "Enqueue Message.vi"("error in (no error)"=w382, "Message"="Start Loops", "Message Queue"=w383) -> ("error out"=w384:errorcluster)  [unwired: 7 in, 1 out]
        n129 = Merge Errors(w384) -> (w378:errorcluster)
        n130 = Unbundle By Name(w377) -> ("Agitator Module Config.Process Name"=w381:string)
        n131 = Concatenate Strings(w381, " Start" ("text")) -> (w379:string)
        n132 = call "Write to Log File.vi"("error in"=w378, "text"=w379) -> ()  [unwired: 9 in, 1 out]
      }
      frame "Sequence Start" {
        # "Message Acquisition and Logging loops to start"
        n133 = call-poly "Enqueue Message.vi"("error in (no error)"=w388, "Message"="Broadcast settings", "Message Queue"=w387) -> ("error out"=w395:errorcluster, "dup Message Queue"=w396:refnum<queue>)  [unwired: 7 in]
        n134 = case shown="False" w389 {
          selector: w389 -> [_ w408]
          tunnel: [TRUE w408] -> w390
          tunnel: w395 -> [w406 w409]
          tunnel: w396 -> [w404 _]
          tunnel: [w403 w409] -> w400
          frame False {
            # "Start the loop if it isn't started yet"
            n135 = call-poly "Enqueue Message.vi"("error in (no error)"=w406, "Message"="Start Loops", "Message Queue"=w404) -> ("error out"=w403:errorcluster)  [unwired: 7 in, 1 out]
          }
          frame True {
          }
        }
        n136 = Bundle By Name(cluster=w394, "State"=State_Enum."Measuring") -> (w393:T7)
        n137 = Merge Errors(w400) -> (w391:errorcluster)
        n138 = Unbundle By Name(w393) -> ("Agitator Module Config.Process Name"=w399:string)
        n139 = Concatenate Strings(w399, " Sequence Start" ("text")) -> (w397:string)
        n140 = call "Write to Log File.vi"("error in"=w391, "text"=w397) -> ()  [unwired: 9 in, 1 out]
      }
      frame "Start Loops" {
        # "I'm not sure what we would have multiple Process names in a module for but i'll leave it for now."
        # "Message Acquisition and Logging loops to start"
        # "Start - Enable/Disable buttons appropriately for an acquisition that has started, and update status display."
        n141 = Build Array(w416) -> (w414:refnum<queue>[])
        n142 = Unbundle By Name(w412) -> ("Agitator Module Config.Process Name"=w413:string)
        n143 = for {
          tunnel: w411 -> [w422]
          tunnel: [w421] -> w415 mode=indexing
          tunnel: w414 -> [w420] mode=indexing
          tunnel: w413 -> [w419]
          n144 = call-poly "Enqueue Message.vi"("error in (no error)"=w422, "Message Data"=w419, "Message"="Start", "Message Queue"=w420) -> ("error out"=w421:errorcluster)  [unwired: 6 in, 1 out]
        }
        n145 = Merge Errors(w411, w415) -> (w418:errorcluster)
      }
      frame "Start Log" {
        # "I'm not sure what we would have multiple Process names in a module for but i'll leave it for now."
        # "Message Acquisition and Logging loops to start"
        # "Start - Enable/Disable buttons appropriately for an acquisition that has started, and update status display."
        n146 = Build Array(w434) -> (w432:refnum<queue>[])
        n147 = Unbundle By Name(w426) -> ("Agitator Module Config.Process Name"=w431:string)
        n148 = property class="VI"("Front Panel.Title"=w431) -> ()  [unwired: 2 in, 2 out]
        n149 = for {
          tunnel: w425 -> [w439]
          tunnel: [w438] -> w433 mode=indexing
          tunnel: w432 -> [w437] mode=indexing
          tunnel: w431 -> [w436]
          n150 = call-poly "Enqueue Message.vi"("error in (no error)"=w439, "Message Data"=w436, "Message"="Start Log", "Message Queue"=w437) -> ("error out"=w438:errorcluster)  [unwired: 6 in, 1 out]
        }
        n151 = Merge Errors(w425, w433) -> (w427:errorcluster)
        n152 = Unbundle By Name(w426) -> ("Agitator Module Config.Process Name"=w430:string)
        n153 = Concatenate Strings(w430, " Start Log" ("text")) -> (w428:string)
        n154 = call "Write to Log File.vi"("error in"=w427, "text"=w428) -> ()  [unwired: 9 in, 1 out]
      }
      frame "Stop" {
        # "Stop - Enable/Disable buttons appropriately for an acquisition that has stopped, and update status display."
        n155 = call-poly "Enqueue Message.vi"("error in (no error)"=w451, "Message Data"="Ready..." ("Ready..."), "Message"="Update Status", "Message Queue"=w456) -> ("error out"=w449:errorcluster)  [unwired: 6 in, 1 out]
        n156 = call-poly "Enqueue Message.vi"("error in (no error)"=w449, "Message"="Pause", "Message Queue"=w450) -> ("error out"=w447:errorcluster)  [unwired: 7 in, 1 out]
        n157 = case shown="Default" w452 {
          selector: w452 -> [_ w458]
          tunnel: [UI_State."Waiting for Stop" ("UI State") w458] -> w453
          frame Default {
          }
          frame "Waiting for Exit" {
          }
        }
        n158 = Merge Errors(w447) -> (w443:errorcluster)
        n159 = Unbundle By Name(w442) -> ("Agitator Module Config.Process Name"=w446:string)
        n160 = Concatenate Strings(w446, " Stop" ("text")) -> (w444:string)
        n161 = call "Write to Log File.vi"("error in"=w443, "text"=w444) -> ()  [unwired: 9 in, 1 out]
      }
      frame "Update Status" {
        # "Update Display - Convert the message data to a string to display in the Status indicator."
        n162 = Variant To Data(error in=w466, type="", Variant=w465) -> (data=→"Status":string, error out=w463:errorcluster)
        n163 = Merge Errors(w463) -> (w467:errorcluster)
      }
      frame Default {
        # "'Default' case only runs if there is a message that isn't defined in any of the other cases.  Output a programming error."
        n164 = Concatenate Strings("The invalid message string " ("string"), w470, " was received in Scale Module Main" ("string")) -> (w471:string)
        n165 = Bundle By Name(cluster=errorcluster {"status"=TRUE, "code"=1, "source"=""} ("error constant"), "source"=w471) -> (w469:errorcluster)
        n166 = Unbundle By Name(w475) -> ("Agitator Module Config.Process Name"=w478:string)
        n167 = Concatenate Strings(w478, "Invalid Message Recieved" ("text"), w470) -> (w476:string)
        n168 = call "Write to Log File.vi"("error in"=w469, "text"=w476) -> ()  [unwired: 9 in, 1 out]
      }
    }
    n169 = call "Error Handler - Message Handling Loop.vi"("error in (no error)"=w83, "Message Queue"=w81) -> ("dup error in"=w82:errorcluster, "dup Message Queue"=w69:refnum<queue>)  [unwired: 8 in]
  }
  n170 = while {
    tunnel: w22 -> [w491]
    tunnel: [w493] -> w28
    shift-right: [w492] -> w23
    shift-left: w26 -> [w497]
    tunnel: [w490] -> w16
    tunnel: w15 -> [w490]
    tunnel: w12 -> [w489]
    shift-right: [w486] -> _
    shift-left: w6 -> [w485]
    tunnel: [w481] -> w5
    tunnel: [w480] -> w4
    stop <- w496 stop-if-true
    # "Event Handling Loop"
    n171 = call "Dequeue Message.vi"("timeout in ms (-1)"=50, "Message Queue"=w489) -> ("error out"=w482:errorcluster, "Message Data"=w487:variant, "Message"=w488:string, "dup Message Queue"=w483:refnum<queue>)  [unwired: 6 in]
    n172 = Flush Queue(queue=w483, error in (no error)=w482) -> (queue out=w480:refnum<queue>)  [unwired: 2 out]
    n173 = case "Display Update" shown="\"Update\"" w488 {
      tunnel: w487 -> [_ w504]
      tunnel: [w498 w502] -> w486
      tunnel: w485 -> [w498 _]
      frame "False", Default {
      }
      frame "Update" {
        w501 = T13 {"Agitator On?"=enum."Off", "Agitator RPM Value"=0.0, "Cycle Period"=500.0}  # AM Display
        n174 = Variant To Data(type=w501, Variant=w504) -> (data=w503:T13)  [unwired: 1 in, 1 out]
        n175 = Unbundle By Name(w503) -> ("Agitator On?"=w499:T14, "Agitator RPM Value"=→"RPM":dbl, "Cycle Period"=w502:dbl)
        n176 = property on="Image Ring" class="Ring (strict)"("Value"=w499) -> ()  [unwired: 2 in, 2 out]
      }
    }
    n177 = event shown="[1] Panel Resize" {
      selector: w497 -> [_ _ _ _ _ _ _]
      dyn-events: [_ _ _ _ _ _ _] -> w492
      timeout: w486 -> [_ _ _ _ _ _ _]
      tunnel: [_ _ _ TRUE ("Discard?") TRUE ("Discard?") _ _] -> w496
      tunnel: w491 -> [w505 w513 w516 w520 w526 w531 w541]
      tunnel: [_ _ w514 w525 _ w533 _] -> w494
      tunnel: [w505 w513 w515 w523 w526 w532 w541] -> w495
      event Timeout {
        n178 = event-data() -> ()  [unwired: 1 in, 1 out]
      }
      event Panel Resize {
        n179 = event-data() -> ("NewBnds"=w508:T15)  [unwired: 1 in]
        n180 = local read "Original Width"() -> (w509:u32)
        n181 = call "Front End Resize.vi"("Starting Font"=6.0, "Area to Font Division"=400.0, "Original Text Box Width"=64, "NewBnds"=w508, "Original Panel Width"=w509) -> ("New Text Box Width"=w507:u64, "New Font Size"=w506:dbl)  [unwired: 5 in]
        n182 = property on="RPM" class="DigNum (strict)"("NumText.FontSize"=w506) -> ()  [unwired: 2 in, 2 out]
        n183 = property on="RPM" class="DigNum (strict)"("Text Width"=w507) -> ()  [unwired: 2 in, 2 out]
        n184 = property on="RPM" class="DigNum (strict)"("Label.FontSize"=w506) -> ()  [unwired: 2 in, 2 out]
      }
      event Panel Close? {
        w517 = TRUE  # Priority Message
        n185 = event-data() -> ()  [unwired: 1 in, 1 out]
        n186 = call-poly "Enqueue Message.vi"("Priority Message? (F)"=w517, "Message"="Confirm Quit", "Message Queue"=w516) -> ("error out"=w514:errorcluster, "dup Message Queue"=w515:refnum<queue>)  [unwired: 7 in]
        n187 = event-data("Discard?"=TRUE) -> ()  [unwired: 1 in, 1 out]
      }
      event "Exit": Value Change {
        w521 = TRUE  # Priority Message
        # "The UI Message Loop handles sending the Exit message to other loops."
        n188 = event-data() -> ()  [unwired: 1 in, 1 out]
        n189 = call-poly "Enqueue Message.vi"("Priority Message? (F)"=w521, "Message"="Exit", "Message Queue"=w520) -> ("error out"=w525:errorcluster, "dup Message Queue"=w523:refnum<queue>)  [unwired: 7 in]
      }
      event User Event {
        # "The Message Handling Loop processed an \"Exit\" message, which fired this event to stop the Event Handling Loop."
        n190 = event-data() -> ()  [unwired: 1 in, 1 out]
        n191 = local write "Status"("Exit" ("Exit String")) -> ()
      }
      event "Settings Button": Mouse Down {
        # "Allow debugging during run with a ctrl click"
        n192 = event-data() -> ("PlatMods"=w530:T16)  [unwired: 1 in]
        n193 = Unbundle By Name(w530) -> ("Ctrl"=w529:bool)
        n194 = case shown="False" w529 {
          tunnel: [w537 w538] -> w533
          tunnel: [w536 w539] -> w532
          tunnel: w531 -> [w535 w539]
          frame False {
            n195 = call-poly "Enqueue Message.vi"("Message"="Launch Settings Dialog", "Message Queue"=w535) -> ("error out"=w537:errorcluster, "dup Message Queue"=w536:refnum<queue>)  [unwired: 8 in]
          }
          frame True {
            n196 = property class="VI"("BDWin.Open"=TRUE ("Block Diagram Window:Open")) -> (error out=w538:errorcluster)  [unwired: 2 in, 1 out]
          }
        }
      }
      event Key Down {
        n197 = event-data() -> ("ScanCode"=→"ScanCode":i16)  [unwired: 1 in]
      }
    }
    n198 = call "Error Handler - Event Handling Loop.vi"("error in (no error)"=w494, "Message Queue"=w495) -> ("dup error in"=w493:errorcluster, "dup Message Queue"=w481:refnum<queue>)  [unwired: 8 in]
  }
  n199 = call "Main Loop.vi"("error in (no error)"=w11, "Chart Notifier"=w17, "Message Queues"=w10) -> ("error out"=w18:errorcluster)  [unwired: 8 in]
  n200 = Unregister For Events(event registration refnum=w23, error in=w28) -> (error out=w24:errorcluster)
  n201 = Close Reference(reference=w16) -> ()  [unwired: 1 in, 1 out]
  n202 = Merge Errors(w24, w29, w11, w18) -> (w27:errorcluster)
  n203 = Release Queue(queue=w5) -> ()  [unwired: 2 in, 3 out]
  n204 = Release Queue(queue=w4) -> ()  [unwired: 2 in, 3 out]
  n205 = Release Queue(queue=w3) -> ()  [unwired: 2 in, 3 out]
  n206 = call "Destroy User Event - Stop.vi"("error in (no error)"=w27, "User Event - Stop"=w25) -> ("error out"=w7:errorcluster)  [unwired: 9 in]
  n207 = flat-sequence {
    tunnel: w7 -> [_]
    frame #0 {
      n208 = invoke class="VI" method="FP.Close"() -> ()  [unwired: 3 in, 3 out]
    }
  }
